vi "WaferImageTest.vi"() -> ()   [LabVIEW 2012]
uses:
  Controls/Waferimage.ctl
  Controls/MapPOS.ctl
  Controls/TestArea.ctl
panel:
  in  "Area":T1
  out "Wafer Out":T2
  in  "Enum":enum16{"Mark", "Clear All"}(ring)
  out "error out":errorcluster
  in  "error in (no error)":errorcluster
  in  "Cluster":T3={"Top"={"left"=208, "top"=106, "right"=218, "bottom"=116}, "CenterC"={"left"=217, "top"=189, "right"=228, "bottom"=200}, "CenterB"={"left"=217, "top"=208, "right"=228, "bottom"=219}, "CenterA"={"left"=199, "top"=208, "right"=209, "bottom"=219}, "Left"={"left"=103, "top"=199, "right"=114, "bottom"=209}, "Right"={"left"=314, "top"=199, "right"=325, "bottom"=209}}
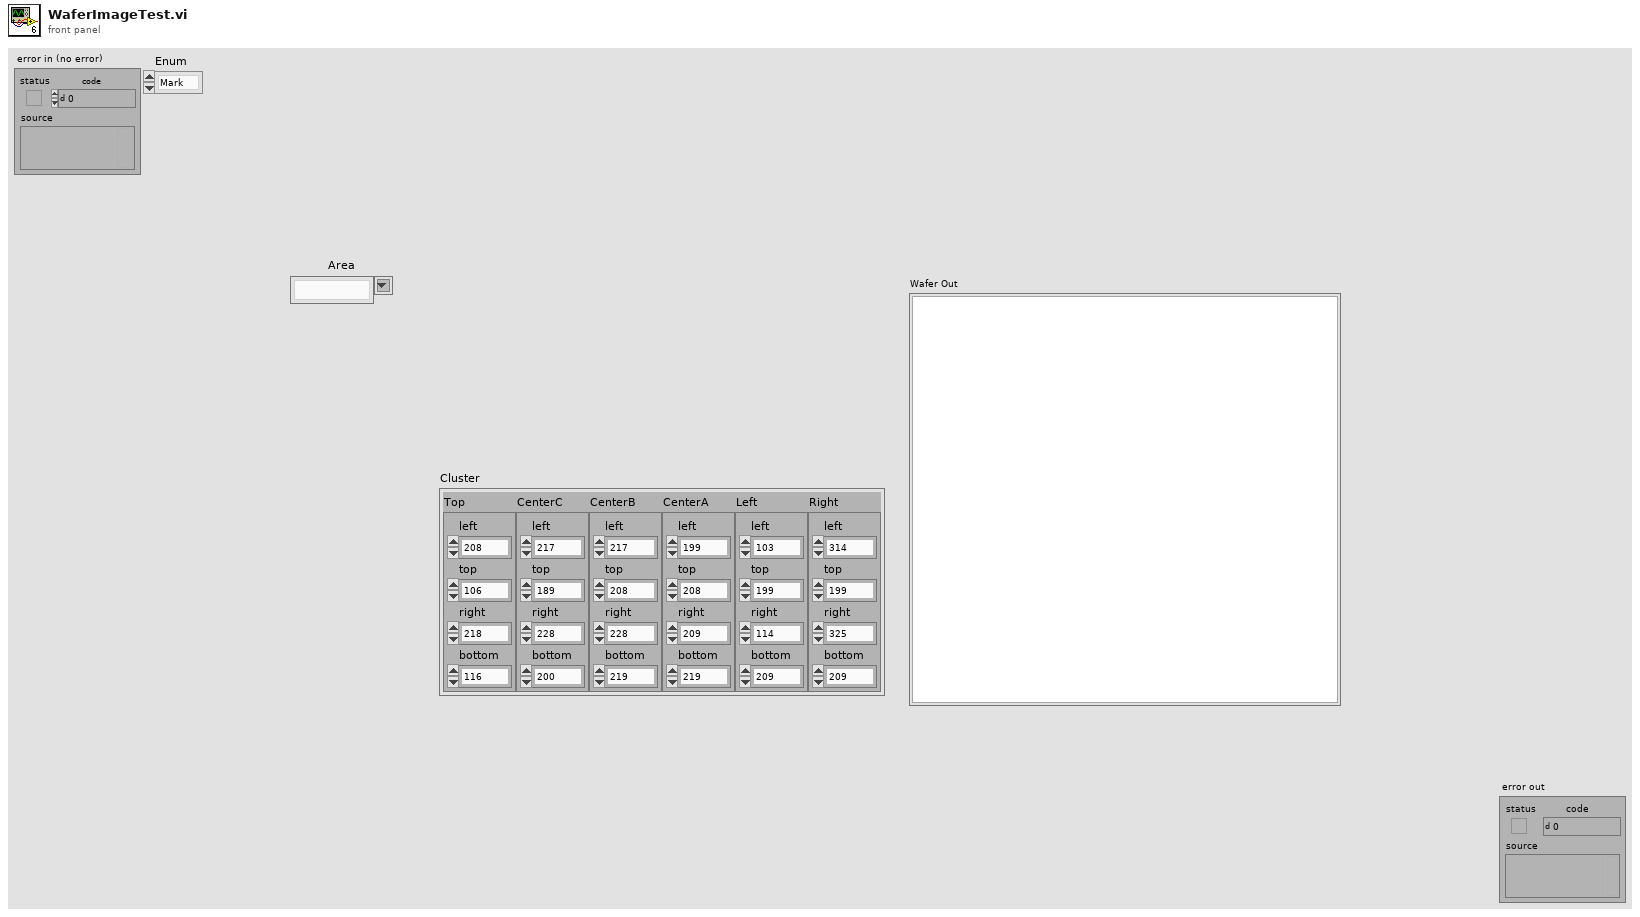
[diagram p1: front panel]
types:
  T1 = typedef "TestArea.ctl" = string
  T2 = typedef "Waferimage.ctl" = picture
  T3 = typedef "MapPOS.ctl" = cluster{"Top":cluster{"left":i16, "top":i16, "right":i16, "bottom":i16}, "CenterC":cluster{"left":i16, "top":i16, "right":i16, "bottom":i16}, "CenterB":cluster{"left":i16, "top":i16, "right":i16, "bottom":i16}, "CenterA":cluster{"left":i16, "top":i16, "right":i16, "bottom":i16}, "Left":cluster{"left":i16, "top":i16, "right":i16, "bottom":i16}, "Right":cluster{"left":i16, "top":i16, "right":i16, "bottom":i16}}
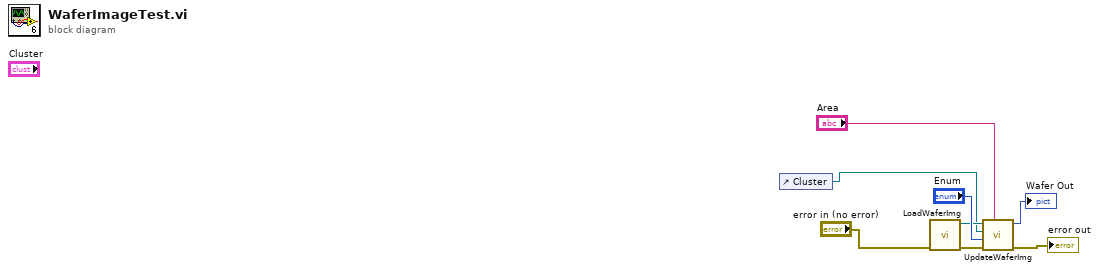
[diagram p0: block diagram]
diagram:
  n1 = control-ref of="Cluster"() -> (w2:refnum<vi>)
  n2 = call "LoadWaferImg.vi"("error in (no error)"="error in (no error)") -> ("error out"=w5:errorcluster, "FrontPanelData out"=w6:refnum<class "EpiWrapper.lvclass">)  [unwired: 9 in]
  n3 = call "UpdateWaferImg.vi"("Area"="Area", "error in (no error)"=w5, "Enum"="Enum", "Cluster 2"=w2, "Wafer in"=w6) -> ("error out"=→"error out":errorcluster, "Wafer Out"=→"Wafer Out":T2)  [unwired: 5 in]
